vi "Pressure_Multiplexer_Sub.vi"(1 "Single Pres Multiplexer":T1) -> (0 "DAQ Error":errorcluster)   [LabVIEW 2021]
uses:
  Device ID port info.ctl
  <vilib>/Instr/_visa.llb/VISA Find Search Mode.ctl
  Sub_vis/Upload Data.ctl
  EnFlo specific/Ctls/Cmd list.ctl
  Globals/Meas_global.vi
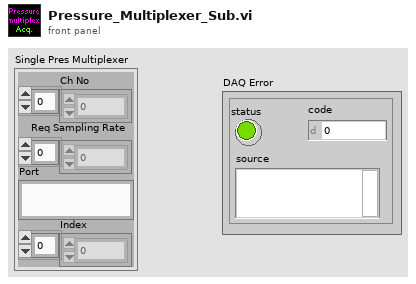
[diagram p1: front panel]
types:
  T1 = typedef "Device ID port info.ctl" = cluster{"Ch No":i16[], "Req Sampling Rate":dbl[], "Port":string, "Index":i32[]}
  T2 = typedef "Setup.ctl" = enum16{"Run Program", "Show Setup", "Save Current Setup", "Setup Front Panel"}
  T3 = typedef "Upload Data.ctl" = enum16{"Voltage Array", "Time Trace Cluster"}
  T4 = typedef "Cmd list.ctl" = string
  T5 = typedef "VISA Find Search Mode.ctl" = u32
  T6 = typedef "Trigger_Mode.ctl" = enum16{"Free Running", "Start on Trigger", "Trigger Every Block", "Trigger Every Sample"}
  T7 = typedef "Data values, Mode 0 (for datalog).ctl" = cluster{"Time Stamp":timestamp, "dt (us)":sgl, "dt_warn":u8, "Pressures":sgl[], "Statuses":u8[]}
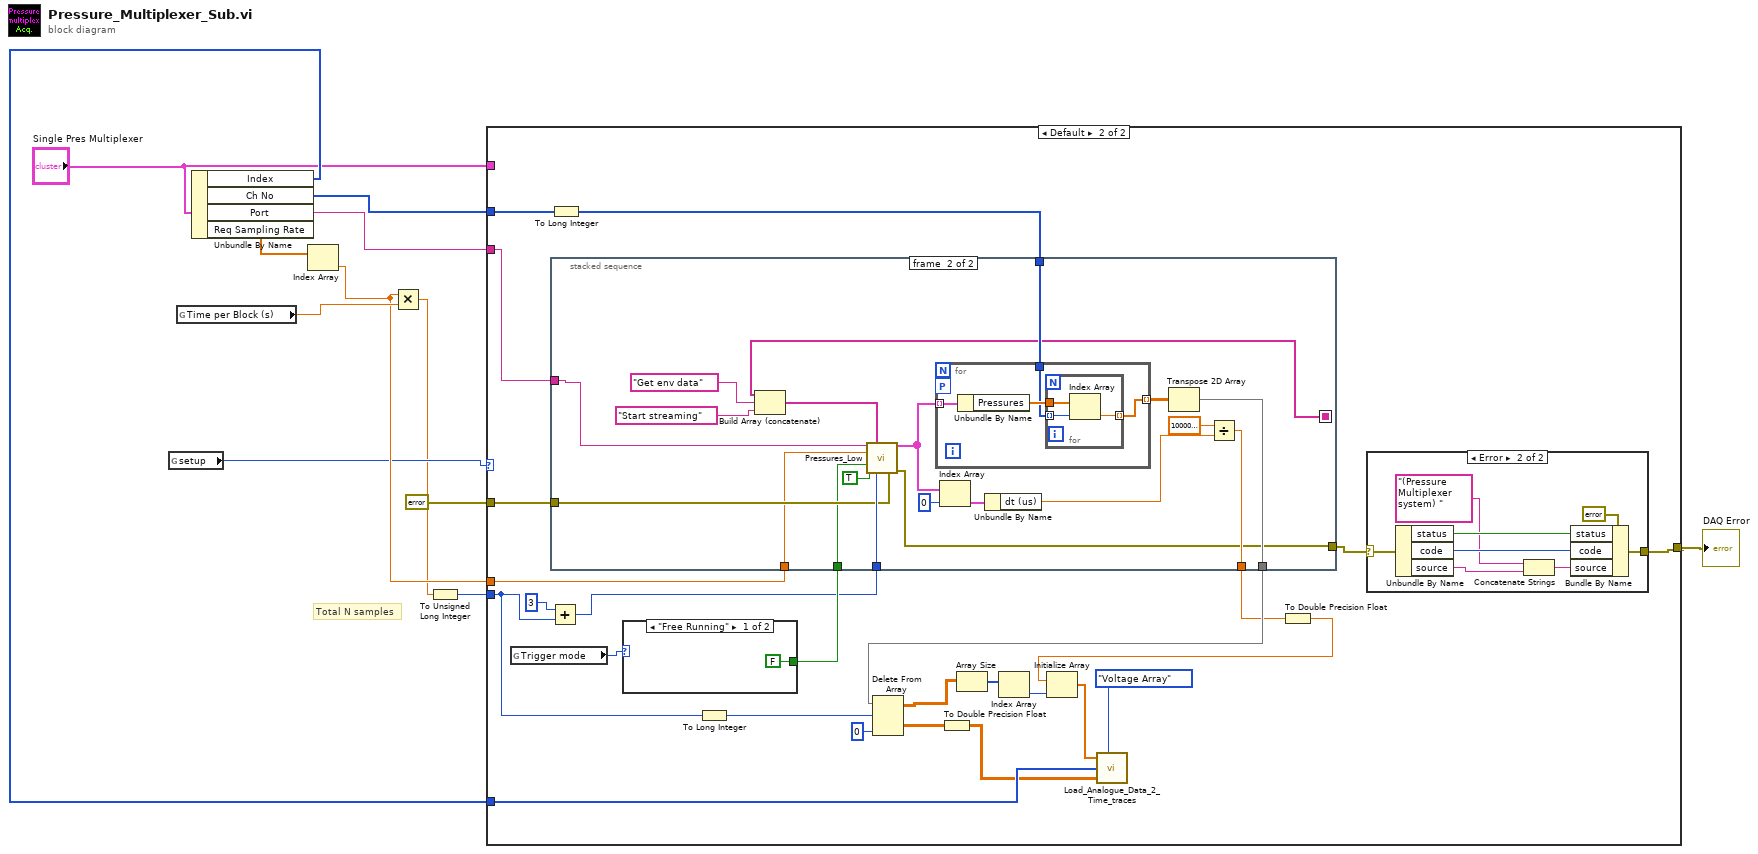
[diagram p0: block diagram]
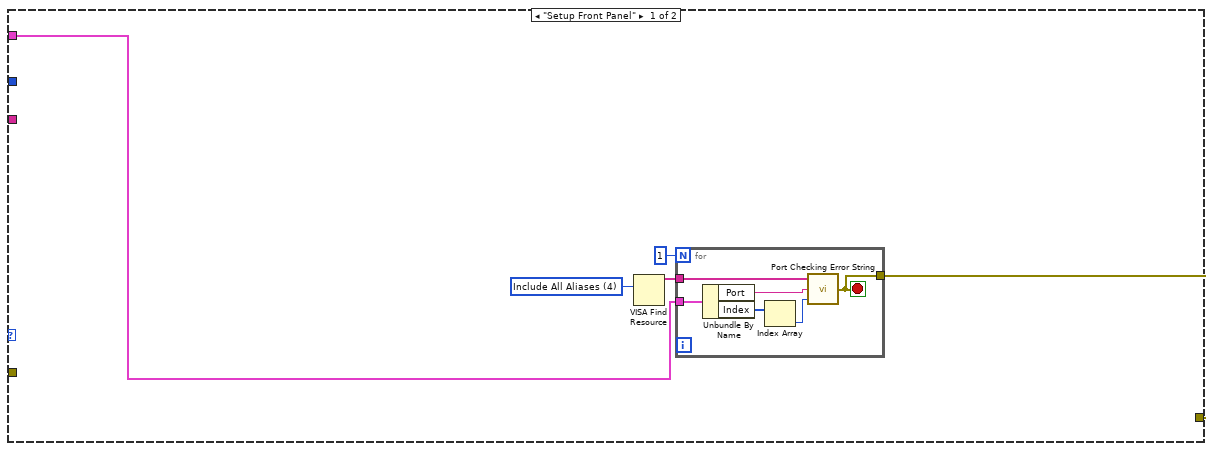
[diagram p2: hidden frame]
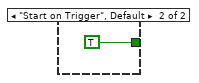
[diagram p3: hidden frame]
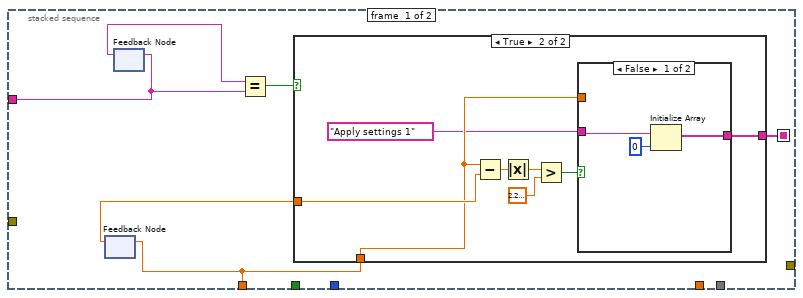
[diagram p4: hidden frame]
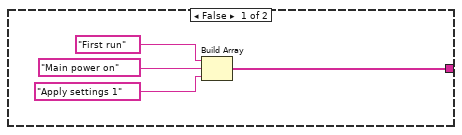
[diagram p5: hidden frame]
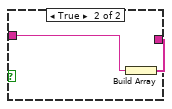
[diagram p6: hidden frame]
diagram:
  # "Total N samples"
  n1 = global read "Meas_global.vi" "setup"() -> (w7:T2)
  n2 = global read "Meas_global.vi" "Time per Block (s)"() -> (w9:dbl)
  n3 = Unbundle By Name("Single Pres Multiplexer") -> ("Index"=w4:i32[], "Ch No"=w3:i16[], "Port"=w6:string, "Req Sampling Rate"=w5:dbl[])
  n4 = Index Array(array=w5) -> (element=w8:dbl)  [unwired: 1 in]
  n5 = Multiply(x=w8, y=w9) -> (x*y=w1:dbl)
  n6 = To Unsigned Long Integer(number=w1) -> (unsigned 32bit integer=w11:u32)
  n7 = case shown="Default" w7 {
    tunnel: [w13 w48] -> w12
    tunnel: w11 -> [_ w24]
    tunnel: errorcluster {"status"=FALSE, "code"=0, "source"=""} ("Error in") -> [_ w45]
    tunnel: w8 -> [_ w30]
    tunnel: w6 -> [_ w31]
    tunnel: w3 -> [_ w44]
    tunnel: w4 -> [_ w43]
    tunnel: "Single Pres Multiplexer" -> [w15 _]
    frame "Setup Front Panel" {
      w16 = T5 4 items=["Canonical Names Only"=0, "Aliases Only"=1, "Include Matching Aliases"=2, "Include All Aliases"=4] ("Search Mode")
      n8 = VISA Find Resource(10:w16) -> (3:w17:string[])  [unwired: 2 in, 2 out]
      n9 = for {
        N: 1 -> [_]
        tunnel: w15 -> [w23]
        tunnel: w17 -> [w19]
        tunnel: [w18] -> w13
        stop <- w18 stop-if-true
        n10 = Unbundle By Name(w23) -> ("Port"=w20:string, "Index"=w22:i32[])
        n11 = Index Array(array=w22) -> (element=w21:i32)  [unwired: 1 in]
        n12 = call "Port Checking Error String.vi"("Ch Index"=w21, "Port"=w20, "Available Ports"=w19) -> ("error out"=w18:errorcluster)  [unwired: 1 in]
      }
    }
    frame Default {
      n13 = global read "Meas_global.vi" "Trigger mode"() -> (w29:T6)
      n14 = Add(x=u32 3, y=w24) -> (x+y=w26:u32)
      n15 = To Long Integer(number=w44) -> (32bit integer=w32:i32[])
      n16 = case shown="\"Free Running\"" w29 {
        tunnel: [FALSE ("Wait for HW trigger") TRUE ("Wait for HW trigger")] -> w28
        frame "Free Running" {
        }
        frame "Start on Trigger", Default {
        }
      }
      n17 = stacked-sequence {
        seq-local: [w52 _] -> [_ w79]
        tunnel: w45 -> [_ w76]
        tunnel: w31 -> [w55 w77]
        tunnel: w30 -> [w51 w75]
        tunnel: [_ w84] -> w33
        tunnel: [_ w87] -> w46
        tunnel: [_ w93] -> w34
        tunnel: w26 -> [_ w83]
        tunnel: w32 -> [_ w82]
        tunnel: w28 -> [_ w74]
        frame #0 {
          n18 = feedback-in #1(w51) -> ()
          n19 = feedback #1() -> (w56:dbl)  [unwired: 1 in]
          n20 = feedback #2() -> (w54:string)  [unwired: 1 in]
          n21 = feedback-in #2(w55) -> ()
          n22 = Equal?(x=w54, y=w55) -> (x = y?=w53:bool)
          n23 = case shown="True" w53 {
            tunnel: w56 -> [_ w64]
            tunnel: w51 -> [_ w63]
            tunnel: [w57 w62] -> w52
            frame False {
              n24 = Build Array(T4 "First run" ("Command"), T4 "Main power on" ("Command"), T4 "Apply settings 1" ("Command")) -> (w57:T4[])
            }
            frame True {
              n25 = Subtract(x=w63, y=w64) -> (x-y=w66:dbl)
              n26 = Absolute Value(x=w66) -> (abs(x)=w67:dbl)
              n27 = Greater?(x=w67, y=2.220446049250313e-16) -> (0:w65:bool)
              n28 = case shown="False" w65 {
                tunnel: w63 -> [_ _]
                tunnel: [w69 w73] -> w62
                tunnel: T4 "Apply settings 1" ("Command") -> [w71 w72]
                frame False {
                  n29 = Initialize Array(w71, 0 ("dimension size")) -> (w69:T4[])
                }
                frame True {
                  n30 = Build Array(w72) -> (w73:T4[])
                }
              }
            }
          }
        }
        frame #1 {
          n31 = Build Array (concatenate)(w79, T4 "Get env data" ("Command"), T4 "Start streaming" ("Command")) -> (w78:T4[])
          n32 = call "Pressures_Low.vi"("Serial port"=w77, "Commands"=w78, "Data rate (Hz)"=w75, "Wait for HW trigger"=w74, "Finite samples"=TRUE, "N samples"=w83, "Error in"=w76) -> ("P data (mode 0)"=w85:T7[], "Error out"=w84:errorcluster)  [unwired: 7 in]
          n33 = for {
            tunnel: [w95] -> w91 mode=indexing
            tunnel: w85 -> [w97] mode=indexing
            workers-P: _ -> [_]
            tunnel: w82 -> [w94]
            n34 = Unbundle By Name(w97) -> ("Pressures"=w96:sgl[])
            n35 = for {
              tunnel: w94 -> [w100] mode=indexing
              tunnel: w96 -> [w99]
              tunnel: [w98] -> w95 mode=indexing
              n36 = Index Array(array=w99, index=w100) -> (element=w98:sgl)
            }
          }
          n37 = Index Array(array=w85, index=0) -> (element=w89:T7)
          n38 = Unbundle By Name(w89) -> ("dt (us)"=w88:sgl)
          n39 = Transpose 2D Array(2D array=w91) -> (transposed array=w87:sgl[][])
          n40 = Divide(x=sgl 1000000.0 ("y"), y=w88) -> (x/y=w93:sgl)
        }
      }
      n41 = To Long Integer(number=w24) -> (32bit integer=w47:i32)
      n42 = Delete From Array(array=w46, length=w47, index (col)=0 ("disabled index (col)")) -> (deleted portion=w41:sgl[][], array with subset deleted=w39:sgl[][])  [unwired: 1 in]
      n43 = To Double Precision Float(number=w41) -> (double precision float=w40:dbl[][])
      n44 = Array Size(array=w39) -> (size(s)=w38:i32[])
      n45 = Index Array(array=w38) -> (element=w37:i32)  [unwired: 1 in]
      n46 = To Double Precision Float(number=w34) -> (double precision float=w42:dbl)
      n47 = Initialize Array(w42, w37) -> (w36:dbl[])
      n48 = call "Load_Analogue_Data_2_Time_traces.vi"("Sampling Rate (Hz)"=w36, "Mode"=Upload_Data."Voltage Array", "Index"=w43, "Voltage Array"=w40) -> ()  [unwired: 3 in]
      n49 = case shown="Error" w33 {
        selector: w33 -> [w101 w102]
        tunnel: [w101 w109] -> w48
        frame No Error {
        }
        frame Error {
          n50 = Unbundle By Name(w102) -> ("status"=w107:bool, "code"=w106:i32, "source"=w105:string)
          n51 = Concatenate Strings("(Pressure Multiplexer system) " ("source"), w105) -> (w103:string)
          n52 = Bundle By Name(cluster=errorcluster {"status"=FALSE, "code"=0, "source"=""} ("DAQ Error"), "status"=w107, "code"=w106, "source"=w103) -> (w109:errorcluster)
        }
      }
    }
  }
  "DAQ Error" <- w12
